vi "random_array_2D.vi"(10 "x":i32=64, 11 "y":i32=64) -> (2 "array":i16[][](array[numeric]))   [LabVIEW 2013]
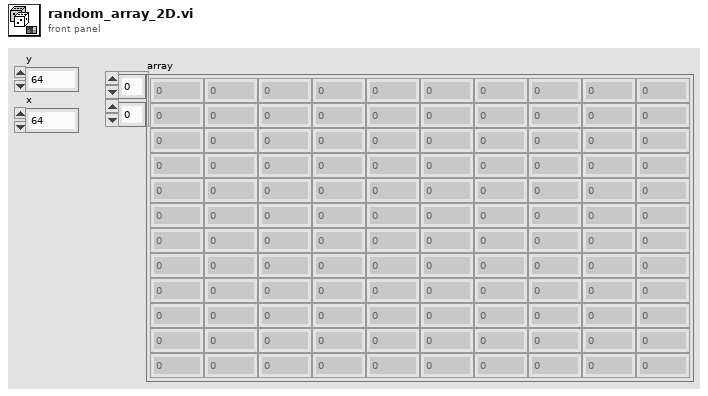
[diagram p1: front panel]
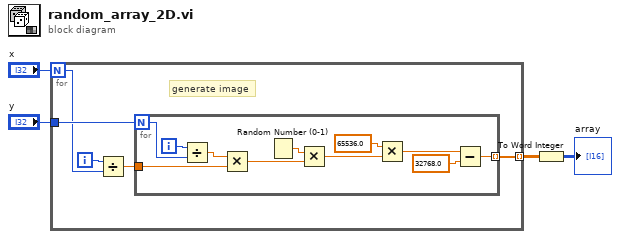
[diagram p0: block diagram]
diagram:
  n1 = for {
    N: "x" -> [w6]
    tunnel: [w9] -> w3 mode=indexing
    tunnel: "y" -> [w8]
    i -> [w7]
    # "generate image"
    n2 = Divide(x=w7, y=w6) -> (x/y=w5:dbl)
    n3 = for {
      N: w8 -> [w15]
      tunnel: [w17] -> w9 mode=indexing
      tunnel: w5 -> [w13]
      i -> [w16]
      n4 = Divide(x=w16, y=w15) -> (x/y=w14:dbl)
      n5 = Multiply(x=w14, y=w13) -> (x*y=w12:dbl)
      n6 = Random Number (0-1)() -> (number: 0 to 1=w11:dbl)
      n7 = Multiply(x=w11, y=w12) -> (x*y=w10:dbl)
      n8 = Multiply(x=65536.0, y=w10) -> (x*y=w19:dbl)
      n9 = Subtract(x=w19, y=32768.0) -> (x-y=w17:dbl)
    }
  }
  n10 = To Word Integer(number=w3) -> (16bit integer=→"array":i16[][])
